vi "set gain sub vi.vi"(2 "error in (no error)":errorcluster, 3 "VISA session":refnum<visa-resource-name>) -> (0 "error out":errorcluster, 1 "dup VISA session":refnum<visa-resource-name>)   [LabVIEW 2009]
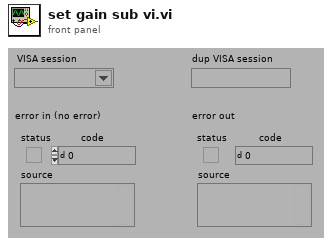
[diagram p1: front panel]
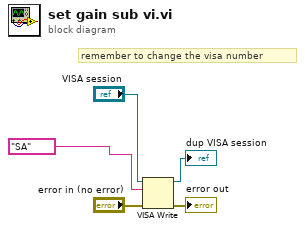
[diagram p0: block diagram]
diagram:
  # "remember to change the visa number"
  n1 = VISA Write(VISA resource name="VISA session", write buffer="SA", error in (no error)="error in (no error)") -> (VISA resource name out=→"dup VISA session":refnum<visa-resource-name>, error out=→"error out":errorcluster)  [unwired: 1 out]
